vi "Remove 2D Array Local Outliers (SGL).vi"(8 "Error In":errorcluster, 9 "Delta (Default: ignore)":sgl=inf, 10 "Percentile (0-100, Default: ignore)":dbl min=0.0 max=100.0, 11 "2D Array in":sgl[][](array[numeric])) -> (0 "Error Out":errorcluster, 3 "2D Array out":sgl[][](array[numeric]))   [LabVIEW 2021, in "Arrays.lvlib"]
uses:
  Arrays.lvlib
  016eccb0-a13b-4e7c-8e90-7371c0dcf4fc.vi
  12e9d21a-84f2-4675-8b0d-3cc4f3b2f5f9.vi
  b07ea3fb-22b5-4eaf-9979-b69b03fc0317.vi
  990491b3-24b3-4a4a-b746-d24a10c52426.vi
  b07ea3fb-22b5-4eaf-9979-b69b03fc0317.vi/3663a709-d1bc-4b7c-975a-3a90df5366f4.vi
  <vilib>/Comparison/Less/Less Functor/Less Functor.lvclass
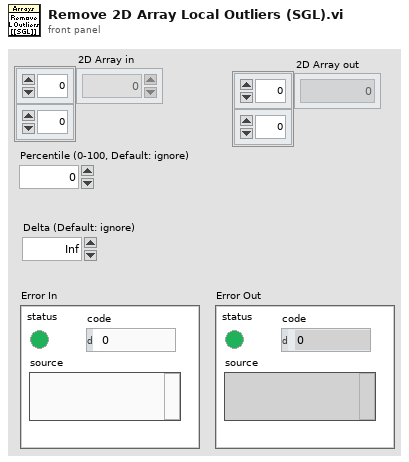
[diagram p1: front panel]
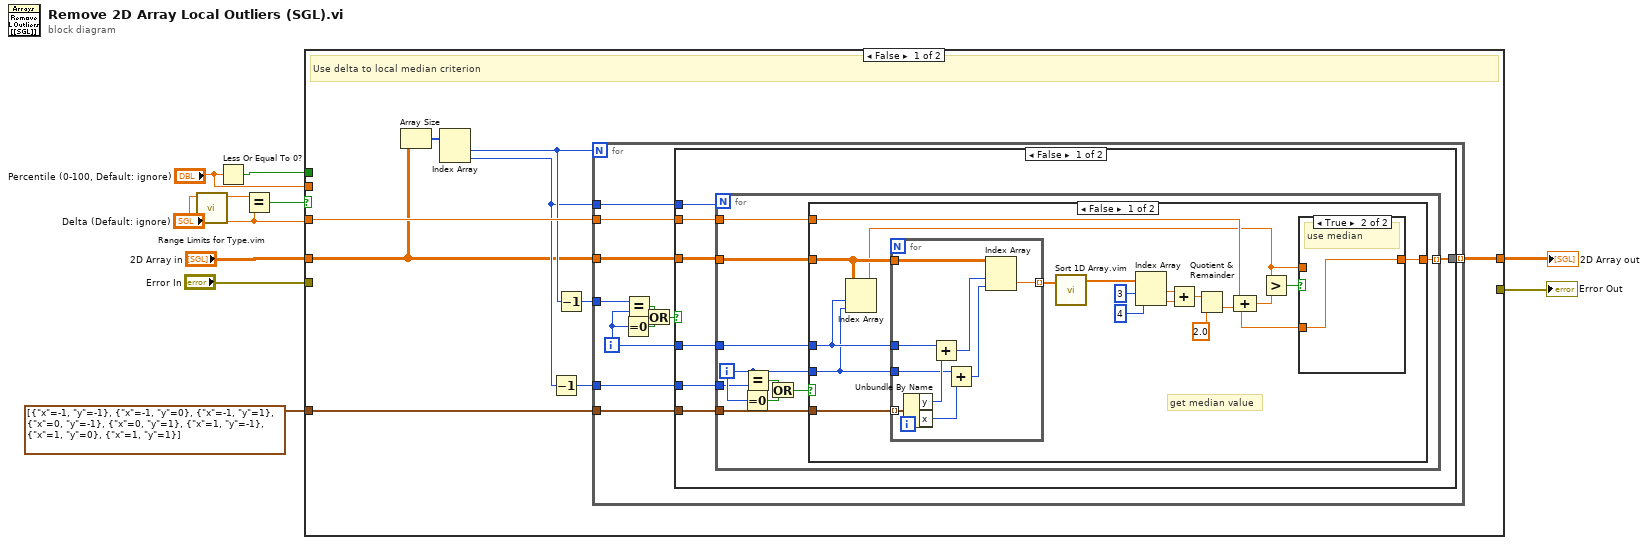
[diagram p0: block diagram]
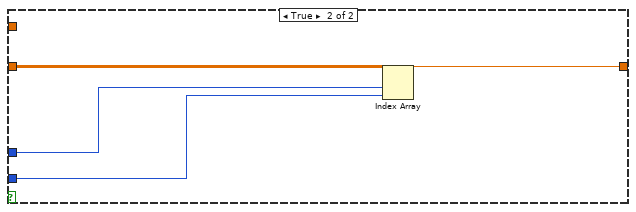
[diagram p3: hidden frame]
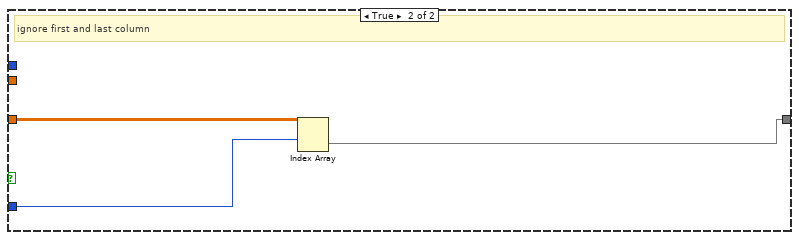
[diagram p4: hidden frame]
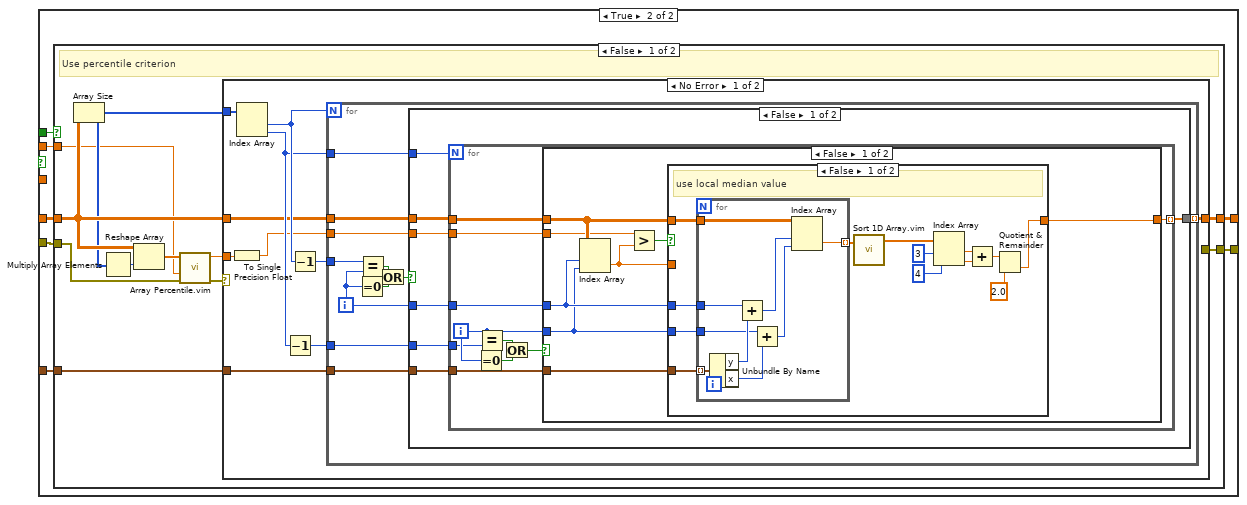
[diagram p5: hidden frame]
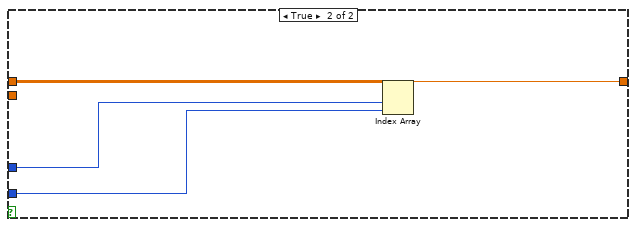
[diagram p7: hidden frame]
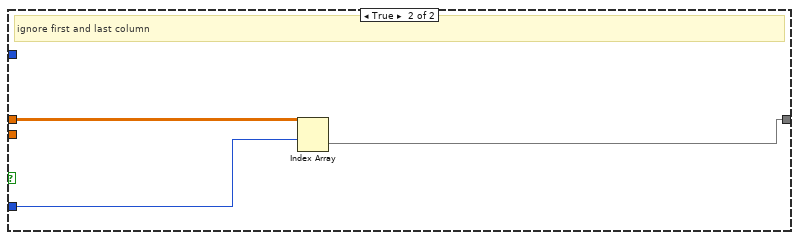
[diagram p8: hidden frame]
diagram:
  n1 = call "Range Limits for Type.vim"("type"="Delta (Default: ignore)") -> ("maximum value for type"=w10:sgl)  [unwired: 9 in, 1 out]
  n2 = Less Or Equal To 0?(x="Percentile (0-100, Default: ignore)") -> (x <= 0?=w8:bool)
  n3 = Equal?(x=w10, y="Delta (Default: ignore)") -> (x = y?=w9:bool)
  n4 = case shown="False" w9 {
    tunnel: "2D Array in" -> [w12 w88]
    tunnel: cluster{"x":i32, "y":i32}[] [{"x"=-1, "y"=-1}, {"x"=-1, "y"=0}, {"x"=-1, "y"=1}, {"x"=0, "y"=-1}, {"x"=0, "y"=1}, {"x"=1, "y"=-1}, {"x"=1, "y"=0}, {"x"=1, "y"=1}] -> [w19 w90]
    tunnel: "Delta (Default: ignore)" -> [w18 _]
    tunnel: [w17 w89] -> w2
    tunnel: w8 -> [_ w87]
    tunnel: "Percentile (0-100, Default: ignore)" -> [_ w84]
    tunnel: "Error In" -> [_ w86]
    tunnel: [_ w85] -> w3
    frame False {
      # "Use delta to local median criterion"
      n5 = Array Size(array=w12) -> (size(s)=w11:i32[])
      n6 = Index Array(array=w11) -> (element #1=w16:i32, element #2=w14:i32)  [unwired: 2 in]
      n7 = Decrement(x=w14) -> (x-1=w13:i32)
      n8 = Decrement(x=w16) -> (x-1=w15:i32)
      n9 = for {
        N: w16 -> [_]
        tunnel: w12 -> [w30]
        tunnel: w19 -> [w29]
        tunnel: w18 -> [w28]
        tunnel: [w27] -> w17 mode=indexing
        tunnel: w14 -> [w26]
        tunnel: w15 -> [w24]
        tunnel: w13 -> [w20]
        i -> [w25]
        n10 = Equal To 0?(x=w25) -> (x = 0?=w22:bool)
        n11 = Equal?(x=w24, y=w25) -> (x = y?=w23:bool)
        n12 = Or(x=w23, y=w22) -> (x .or. y?=w21:bool)
        n13 = case shown="False" w21 {
          tunnel: w30 -> [w37 w83]
          tunnel: w29 -> [w36 _]
          tunnel: w28 -> [w35 _]
          tunnel: [w34 w81] -> w27
          tunnel: w26 -> [w33 _]
          tunnel: w25 -> [w31 w82]
          tunnel: w20 -> [w32 _]
          frame False {
            n14 = for {
              N: w33 -> [_]
              tunnel: w31 -> [w45]
              tunnel: w37 -> [w46]
              tunnel: w36 -> [w47]
              tunnel: w35 -> [w44]
              tunnel: [w43] -> w34 mode=indexing
              tunnel: w32 -> [w39]
              i -> [w40]
              n15 = Equal To 0?(x=w40) -> (x = 0?=w42:bool)
              n16 = Equal?(x=w40, y=w39) -> (x = y?=w41:bool)
              n17 = Or(x=w41, y=w42) -> (x .or. y?=w38:bool)
              n18 = case shown="False" w38 {
                tunnel: w47 -> [w65 _]
                tunnel: w46 -> [w56 w80]
                tunnel: w45 -> [w55 w79]
                tunnel: w44 -> [w52 _]
                tunnel: [w49 w77] -> w43
                tunnel: w40 -> [w54 w78]
                frame False {
                  # "get median value"
                  n19 = Index Array(array=w56, index (row)=w55, index (col)=w54) -> (element=w48:sgl)
                  n20 = for {
                    tunnel: w56 -> [w69]
                    tunnel: w65 -> [w74] mode=indexing
                    tunnel: w55 -> [w73]
                    tunnel: w54 -> [w71]
                    tunnel: [w66] -> w64 mode=indexing
                    n21 = Unbundle By Name(w74) -> ("y"=w72:i32, "x"=w70:i32)
                    n22 = Add(x=w73, y=w72) -> (x+y=w68:i32)
                    n23 = Add(x=w71, y=w70) -> (x+y=w67:i32)
                    n24 = Index Array(array=w69, index (row)=w68, index (col)=w67) -> (element=w66:sgl)
                  }
                  n25 = call "Sort 1D Array.vim"("unsorted array"=w64) -> ("sorted array"=w63:sgl[])  [unwired: 10 in]
                  n26 = Index Array(array=w63, index #1=3 ("index"), index #2=4 ("index")) -> (element #1=w60:sgl, element #2=w59:sgl)
                  n27 = Add(x=w60, y=w59) -> (x+y=w58:sgl)
                  n28 = Quotient & Remainder(x=w58, y=sgl 2.0) -> (floor(x/y)=w50:sgl)  [unwired: 1 out]
                  n29 = Compound Arithmetic op=ADD(w52, w50) -> (w53:sgl)
                  n30 = Greater?(x=w48, y=w53) -> (0:w51:bool)
                  n31 = case shown="True" w51 {
                    tunnel: w50 -> [_ w76]
                    tunnel: w48 -> [w75 _]
                    tunnel: [w75 w76] -> w49
                    frame False {
                      # "keep"
                    }
                    frame True {
                      # "use median"
                    }
                  }
                }
                frame True {
                  # "ignore first and last row"
                  n32 = Index Array(array=w80, index (row)=w79, index (col)=w78) -> (element=w77:sgl)
                }
              }
            }
          }
          frame True {
            # "ignore first and last column"
            n33 = Index Array(array=w83, index (row)=w82) -> (element=w81:sgl[])  [unwired: 1 in]
          }
        }
      }
    }
    frame True {
      n34 = case shown="False" w87 {
        tunnel: w90 -> [w101 _]
        tunnel: [w100 w180] -> w89
        tunnel: w88 -> [w97 w180]
        tunnel: w86 -> [w95 _]
        tunnel: [w93 _] -> w85
        tunnel: w84 -> [w91 _]
        frame False {
          # "Use percentile criterion"
          n35 = Array Size(array=w97) -> (size(s)=w96:i32[])
          n36 = Multiply Array Elements(1:w96) -> (0:w99:i32)
          n37 = Reshape Array(w97, w99) -> (w98:sgl[])
          n38 = call "Array Percentile.vim"("Error In"=w95, "Percentile (0-100)"=w91, "Array"=w98) -> ("Error Out"=w94:errorcluster, "Percentile Value"=w92:sgl)  [unwired: 7 in]
          n39 = case shown="No Error" w94 {
            selector: w94 -> [_ w178]
            tunnel: w101 -> [w111 _]
            tunnel: [w110 w179] -> w100
            tunnel: w97 -> [w105 w179]
            tunnel: w96 -> [w104 _]
            tunnel: [_ w178] -> w93
            tunnel: w92 -> [w103 _]
            frame No Error {
              n40 = To Single Precision Float(number=w103) -> (single precision float=w102:sgl)
              n41 = Index Array(array=w104) -> (element #1=w109:i32, element #2=w107:i32)  [unwired: 2 in]
              n42 = Decrement(x=w107) -> (x-1=w106:i32)
              n43 = Decrement(x=w109) -> (x-1=w108:i32)
              n44 = for {
                N: w109 -> [_]
                tunnel: w105 -> [w122]
                tunnel: w111 -> [w121]
                tunnel: [w120] -> w110 mode=indexing
                tunnel: w107 -> [w119]
                tunnel: w108 -> [w117]
                tunnel: w106 -> [w113]
                tunnel: w102 -> [w112]
                i -> [w118]
                n45 = Equal To 0?(x=w118) -> (x = 0?=w115:bool)
                n46 = Equal?(x=w117, y=w118) -> (x = y?=w116:bool)
                n47 = Or(x=w116, y=w115) -> (x .or. y?=w114:bool)
                n48 = case shown="False" w114 {
                  tunnel: w122 -> [w129 w177]
                  tunnel: w121 -> [w128 _]
                  tunnel: [w127 w175] -> w120
                  tunnel: w119 -> [w126 _]
                  tunnel: w118 -> [w124 w176]
                  tunnel: w113 -> [w125 _]
                  tunnel: w112 -> [w123 _]
                  frame False {
                    n49 = for {
                      N: w126 -> [_]
                      tunnel: w124 -> [w137]
                      tunnel: w129 -> [w138]
                      tunnel: w128 -> [w139]
                      tunnel: [w136] -> w127 mode=indexing
                      tunnel: w125 -> [w132]
                      tunnel: w123 -> [w130]
                      i -> [w133]
                      n50 = Equal To 0?(x=w133) -> (x = 0?=w135:bool)
                      n51 = Equal?(x=w133, y=w132) -> (x = y?=w134:bool)
                      n52 = Or(x=w134, y=w135) -> (x .or. y?=w131:bool)
                      n53 = case shown="False" w131 {
                        tunnel: w139 -> [w147 _]
                        tunnel: w138 -> [w146 w174]
                        tunnel: w137 -> [w145 w173]
                        tunnel: [w141 w171] -> w136
                        tunnel: w133 -> [w144 w172]
                        tunnel: w130 -> [w143 _]
                        frame False {
                          n54 = Index Array(array=w146, index (row)=w145, index (col)=w144) -> (element=w140:sgl)
                          n55 = Greater?(x=w143, y=w140) -> (0:w142:bool)
                          n56 = case shown="False" w142 {
                            tunnel: w147 -> [w160 _]
                            tunnel: w146 -> [w151 _]
                            tunnel: w145 -> [w150 _]
                            tunnel: w144 -> [w149 _]
                            tunnel: [w148 w170] -> w141
                            tunnel: w140 -> [_ w170]
                            frame False {
                              # "use local median value"
                              n57 = for {
                                tunnel: w151 -> [w164]
                                tunnel: w160 -> [w169] mode=indexing
                                tunnel: w150 -> [w168]
                                tunnel: w149 -> [w166]
                                tunnel: [w161] -> w159 mode=indexing
                                n58 = Unbundle By Name(w169) -> ("y"=w167:i32, "x"=w165:i32)
                                n59 = Add(x=w168, y=w167) -> (x+y=w163:i32)
                                n60 = Add(x=w166, y=w165) -> (x+y=w162:i32)
                                n61 = Index Array(array=w164, index (row)=w163, index (col)=w162) -> (element=w161:sgl)
                              }
                              n62 = call "Sort 1D Array.vim"("unsorted array"=w159) -> ("sorted array"=w158:sgl[])  [unwired: 10 in]
                              n63 = Index Array(array=w158, index #1=3 ("index"), index #2=4 ("index")) -> (element #1=w155:sgl, element #2=w154:sgl)
                              n64 = Add(x=w155, y=w154) -> (x+y=w153:sgl)
                              n65 = Quotient & Remainder(x=w153, y=sgl 2.0) -> (floor(x/y)=w148:sgl)  [unwired: 1 out]
                            }
                            frame True {
                              # "keep value"
                            }
                          }
                        }
                        frame True {
                          # "ignore first and last row"
                          n66 = Index Array(array=w174, index (row)=w173, index (col)=w172) -> (element=w171:sgl)
                        }
                      }
                    }
                  }
                  frame True {
                    # "ignore first and last column"
                    n67 = Index Array(array=w177, index (row)=w176) -> (element=w175:sgl[])  [unwired: 1 in]
                  }
                }
              }
            }
            frame Error {
            }
          }
        }
        frame True {
          # "do nothing"
        }
      }
    }
  }
  "Error Out" <- w3
  "2D Array out" <- w2
